vi "lab2_2.vi"() -> ()   [LabVIEW 2026]
panel:
  in  "Cluster":cluster{"Name":string, "Age":dbl, "Gender":bool}
  out "Boolean array":bool[](array[boolean])
  in  "String 2":string
  in  "String":string
  in  "Array 6":bool[][](array[boolean])
  in  "Array 5":bool[][](array[boolean])
  out "Boolean 2":bool
  in  "Boolean":bool
  in  "Array 4":dbl[][](array[numeric])
  in  "Array 3":dbl[][](array[numeric])
  in  "Array 2":dbl[](array[numeric])
  in  "Array":dbl[](array[numeric])
  out "Numeric 4":dbl
  in  "Numeric 3":i8
  out "Numeric 2":dbl
  in  "Numeric":dbl
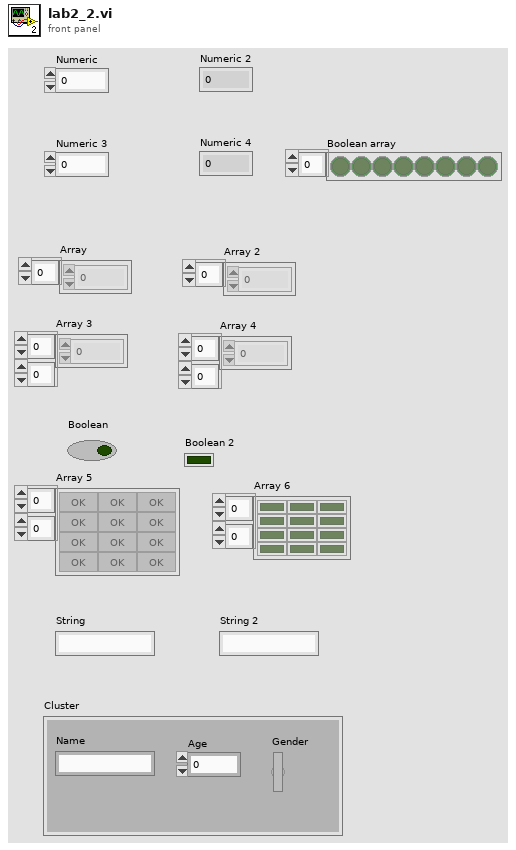
[diagram p1: front panel]
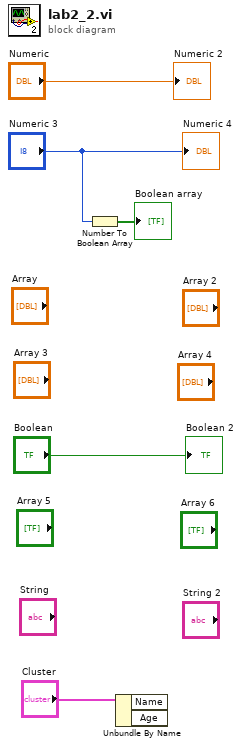
[diagram p0: block diagram]
diagram:
  n1 = Number To Boolean Array(number="Numeric 3") -> (Boolean array=→"Boolean array":bool[])
  n2 = Unbundle By Name("Cluster") -> ()  [unwired: 2 out]
  "Numeric 2" <- "Numeric"
  "Numeric 4" <- "Numeric 3"
  "Boolean 2" <- "Boolean"
